vi "Add ExpGroup.vi"(8 "error in (no error)":errorcluster, 9 "folder of the day":string="no name", 10 "Group title":string, 11 "Control-Client in":refnum<class "Control-Client.lvclass">) -> (0 "error out":errorcluster, 3 "Control-Client out":refnum<class "Control-Client.lvclass">)   [LabVIEW 2015, in "Control-Client.lvclass"]
uses:
  Control-Client.lvclass
  Experiments/Experiment.lvclass
  Experiments/Experiments_group.lvclass
  Control-Client.lvclass/Control-Client.ctl
  Erase color.vi
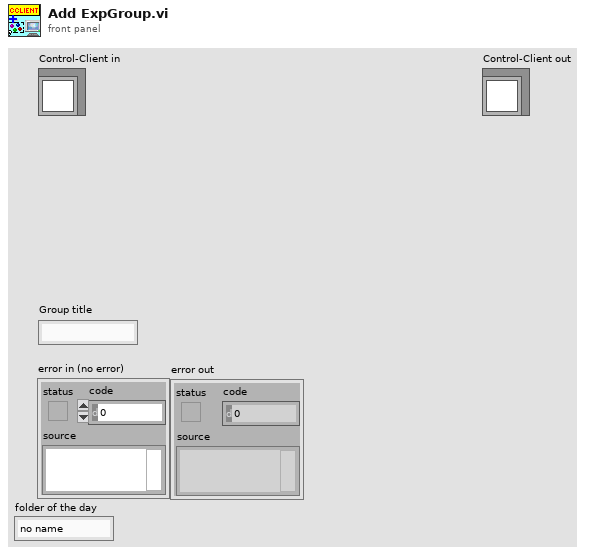
[diagram p1: front panel]
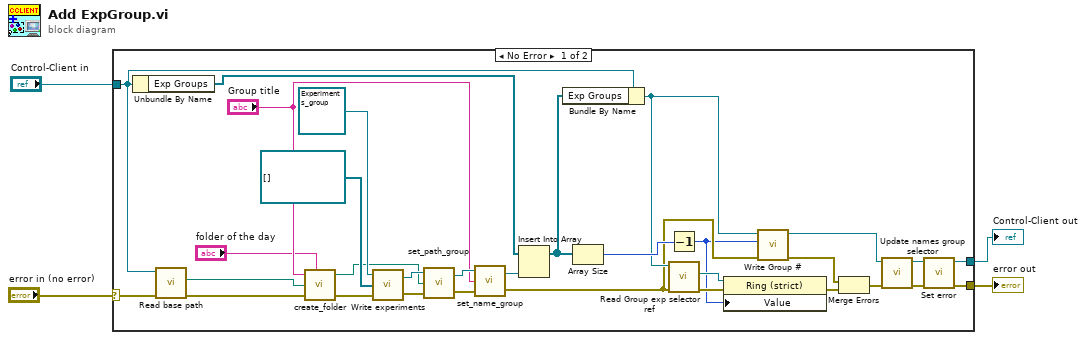
[diagram p0: block diagram]
diagram:
  n1 = case shown="No Error" "error in (no error)" {
    selector: "error in (no error)" -> [w29 w37]
    tunnel: [w8 w37] -> w3
    tunnel: [w7 w36] -> w1
    tunnel: "Control-Client in" -> [w17 w36]
    frame No Error {
      n2 = Unbundle By Name(w17) -> ("Exp Groups"=w27:refnum<class "Experiments_group.lvclass">[])
      n3 = call "Read base path.vi"("error in (no error)"=w29, "Control-Client in"=w17) -> ("error out"=w25:errorcluster, "Base path"=w6:path)  [unwired: 7 in, 1 out]
      n4 = call "create_folder.vi"("Name"="Group title", "folder of the day"="folder of the day", "base path"=w6, "error in"=w25) -> ("appended path"=w23:path, "error out"=w26:errorcluster)  [unwired: 4 in]
      n5 = call-dynamic "Write experiments.vi"("error in (no error)"=w26, "Experiments"=refnum<class "Experiment.lvclass">[] [] ("Experiment array"), "Experiments_group.lvclass in"=refnum<class "Experiments_group.lvclass"> refnum ("element")) -> ("error out"=w30:errorcluster, "Experiments_group.lvclass out"=w31:refnum<class "Experiments_group.lvclass">)
      n6 = call-dynamic "set_path_group.vi"("error in (no error)"=w30, "Path"=w23, "Experiments_group.lvclass in"=w31) -> ("error out"=w35:errorcluster, "Experiments_group.lvclass out"=w33:refnum<class "Experiments_group.lvclass">)
      n7 = call-dynamic "set_name_group.vi"("error in (no error)"=w35, "Name"="Group title", "Experiments_group.lvclass in"=w33) -> ("error out"=w13:errorcluster, "Experiments_group.lvclass out"=w34:refnum<class "Experiments_group.lvclass">)
      n8 = Insert Into Array(array=w27, new element=w34) -> (w19:refnum<class "Experiments_group.lvclass">[])  [unwired: 1 in]
      n9 = Bundle By Name(cluster=w17, "Exp Groups"=w19) -> (w16:refnum<class "Control-Client.lvclass">)
      n10 = Array Size(array=w19) -> (size(s)=w18:i32)
      n11 = Decrement(x=w18) -> (x-1=w11:i32)
      n12 = call "Read Group exp selector ref.vi"("error in (no error)"=w13, "Control-Client in"=w16) -> ("error out"=w22:errorcluster, "Group exp selector ref"=w20:refnum<vi>)  [unwired: 7 in, 1 out]
      n13 = property class="Ring (strict)"(reference=w20, error in=w22, "Value"=w11) -> (error out=w21:errorcluster)  [unwired: 1 out]
      n14 = call "Write Group #.vi"("error in (no error)"=w13, "Group #"=w11, "Control-Client in"=w16) -> ("error out"=w14:errorcluster, "Control-Client out"=w15:refnum<class "Control-Client.lvclass">)  [unwired: 7 in]
      n15 = Merge Errors(w14, w21) -> (w12:errorcluster)
      n16 = call "Update names group selector.vi"("error in (no error)"=w12, "Control-Client in"=w15) -> ("error out"=w9:errorcluster, "Control-Client out"=w10:refnum<class "Control-Client.lvclass">)  [unwired: 8 in]
      n17 = call "Set error.vi"("error in (no error)"=w9, "Control-Client in"=w10) -> ("error out"=w8:errorcluster, "Control-Client out"=w7:refnum<class "Control-Client.lvclass">)  [unwired: 8 in]
    }
    frame Error {
    }
  }
  "error out" <- w3
  "Control-Client out" <- w1
